vi "VeriStand Framework.Create.vi"(8 "error in (no error)":errorcluster, 9 "debug mode (F)":bool, 11 "Device Item Ref":T1=18446744073709551615 format="%.0x") -> (0 "error out":errorcluster, 3 "VeriStand Framework out":refnum<class "VeriStand DSF.Framework.lvclass">)   [LabVIEW 2017, in "Data Sharing Custom Device Engine.lvlib" / "VeriStand DSF.Framework.lvclass"]
uses:
  VeriStand DSF.Framework.lvclass
  <vilib>/NI Veristand/Custom Device API/Custom Device Item Ref.ctl
  Builds/Data Sharing Framework/Current/Data Sharing Framework Core/DSF Core.lvlibp/Engine/Classes/Debug/FIFO Flags.lvclass
  Builds/Data Sharing Framework/Current/Data Sharing Framework Core/DSF Core.lvlibp/Engine/Classes/Debug/Debug Flags.lvclass
  VeriStand DSF.Framework.lvclass/VeriStand DSF.Framework.ctl
  Configuration/VeriStand DSF.Framework.Configuration.lvclass
  Builds/Data Sharing Framework/Current/Data Sharing Framework Core/DSF Core.lvlibp/Engine/Classes/Framework/Framework.lvclass
  C:/Builds/Data Sharing Framework/Current/Data Sharing Framework Core/DSF Core.lvlibp/Engine/Classes/Framework/Framework.lvclass
  C:/Builds/Data Sharing Framework/Current/Data Sharing Framework Core/DSF Core.lvlibp/Shared/Classes/Framework/Framework Configuration.lvclass
  <vilib>/NI Veristand/Custom Device API/Custom Device API.lvlib
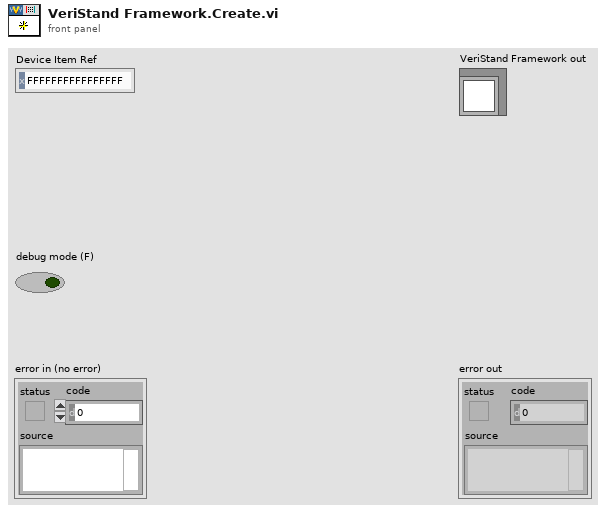
[diagram p1: front panel]
types:
  T1 = typedef "Custom Device API.lvlib/Custom Device Item Ref.ctl" = u64
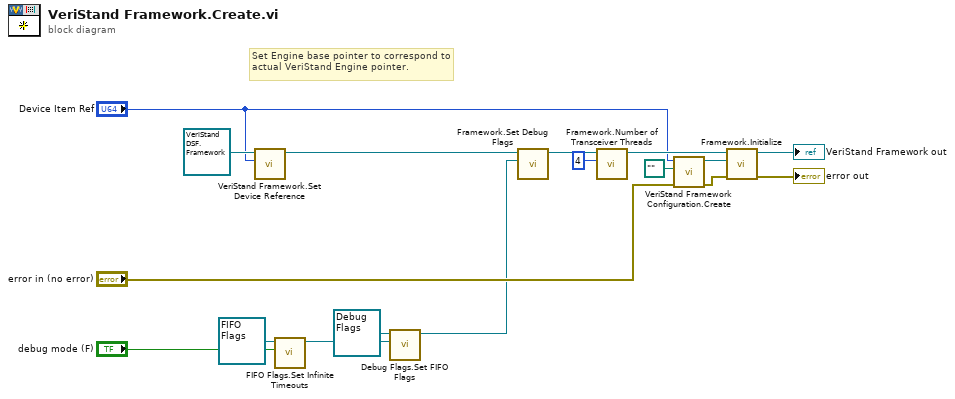
[diagram p0: block diagram]
diagram:
  # "Set Engine base pointer to correspond to actual VeriStand Engine pointer."
  n1 = call "VeriStand Framework.Set Device Reference.vi"("Device Item Ref"="Device Item Ref", "VeriStand Framework in"=refnum<class "VeriStand DSF.Framework.lvclass"> refnum ("VeriStand DSF.Framework.lvclass")) -> ("VeriStand Framework out"=w17:refnum<class "VeriStand DSF.Framework.lvclass">)  [unwired: 9 in]
  n2 = call "FIFO Flags.Set Infinite Timeouts.vi"("infinite timeouts"="debug mode (F)", "FIFO Debug Flags in"=refnum<class "FIFO Flags.lvclass"> refnum) -> ("FIFO Debug Flags out"=w10:refnum<class "FIFO Flags.lvclass">)  [unwired: 9 in]
  n3 = call "Debug Flags.Set FIFO Flags.vi"("FIFO"=w10, "Debug Flags in"=refnum<class "Debug Flags.lvclass"> refnum) -> ("Debug Flags out"=w6:refnum<class "Debug Flags.lvclass">)  [unwired: 9 in]
  n4 = call "Framework.Set Debug Flags.vi"("Debug Flags"=w6, "Framework in"=w17) -> ("Framework out"=w7:refnum<class "VeriStand DSF.Framework.lvclass">)  [unwired: 9 in]
  n5 = call "Framework.Number of Transceiver Threads.vi"("transceiver count"=4, "Framework in"=w7) -> ("Framework out"=w13:refnum<class "VeriStand DSF.Framework.lvclass">)  [unwired: 8 in, 1 out]
  n6 = call "VeriStand Framework Configuration.Create.vi"("error in (no error)"="error in (no error)", "configuration path"=path "", "Device Item Ref"="Device Item Ref") -> ("error out"=w11:errorcluster, "VeriStand Framework Configuration"=w14:refnum<class "VeriStand DSF.Framework.Configuration.lvclass">)  [unwired: 7 in]
  n7 = call "Framework.Initialize.vi"("error in (no error)"=w11, "Framework Configuration"=w14, "Framework type"=w13) -> ("error out"=→"error out":errorcluster, "Framework out"=→"VeriStand Framework out":refnum<class "VeriStand DSF.Framework.lvclass">)  [unwired: 7 in]
